vi "Update Engine Cycle.vi"(8 "error in (no error)":errorcluster, 11 "Mock Framework in":refnum<class "Mock Framework.lvclass">) -> (0 "error out":errorcluster, 3 "Mock Framework out":refnum<class "Mock Framework.lvclass">)   [LabVIEW 2017, in "Mock Framework.lvclass"]
uses:
  Mock Framework.lvclass
  Engine/Classes/Framework/Framework.lvclass
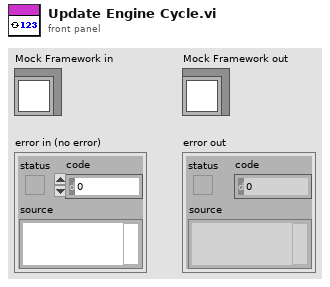
[diagram p1: front panel]
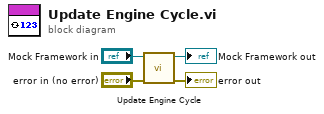
[diagram p0: block diagram]
diagram:
  n1 = call-parent "Update Engine Cycle.vi"("error in (no error)"="error in (no error)", "Framework in"="Mock Framework in") -> ("error out"=→"error out":errorcluster, "Framework out"=→"Mock Framework out":refnum<class "Mock Framework.lvclass">)  [unwired: 8 in]
